vi "inverseKinematicsCode.vi"(8 "Z":dbl, 9 "Y":dbl, 10 "X":dbl) -> (0 "THETA3":dbl, 1 "THETA2":dbl, 2 "THETA1":dbl)   [LabVIEW 2020]
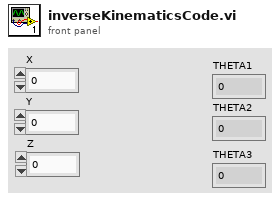
[diagram p1: front panel]
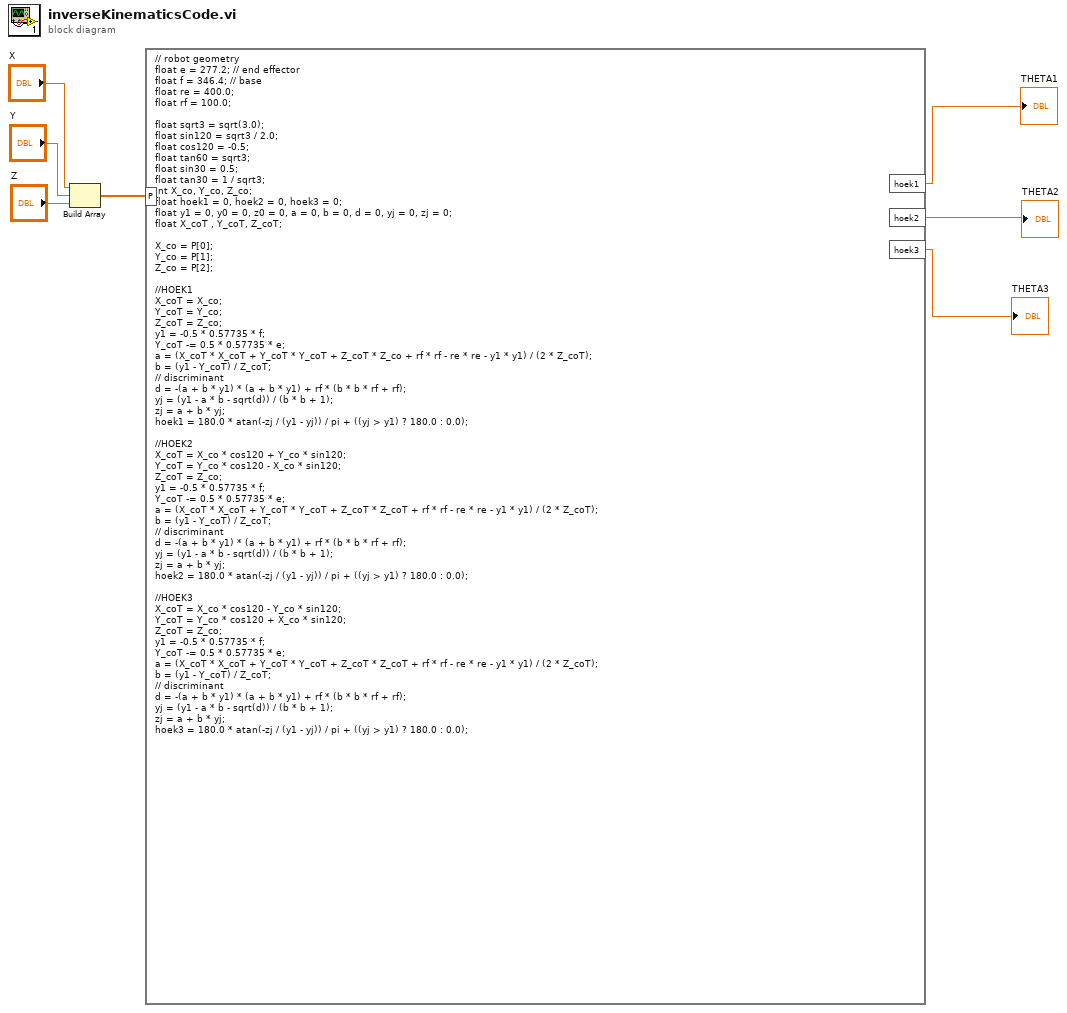
[diagram p0: block diagram]
diagram:
  n1 = Build Array("X", "Y", "Z") -> (w7:dbl[])
  n2 = formula code="// robot geometry\nfloat e = 277.2; // end effector\nfloat f = 346.4; // base\nfloat re = 400.0;\nfloat rf = 100.0;\n\nfloat sqrt3 = sqrt(3.0);\nfloat sin120 = sqrt3 / 2.0;\nfloat cos120 = -0.5;\nfloat tan60 = sqrt3;\nfloat sin30 = 0.5;\nfloat tan30 = 1 / sqrt3;\nint X_co, Y_co, Z_co;\nfloat hoek1 = 0, hoek2 = 0, hoek3 = 0;\nfloat y1 = 0, y0 = 0, z0 = 0, a = 0, b = 0, d = 0, yj = 0, zj = 0;\nfloat X_coT , Y_coT, Z_coT;\n\nX_co = P[0];\nY_co = P[1];\nZ_co = P[2];\n\n//HOEK1\nX_coT = X_co;\nY_coT = Y_co; \nZ_coT = Z_co;\ny1 = -0.5 * 0.57735 * f;\nY_coT -= 0.5 * 0.57735 * e;\na = (X_coT * X_coT + Y_coT * Y_coT + Z_coT * Z_co + rf * rf - re * re - y1 * y1) / (2 * Z_coT);\nb = (y1 - Y_coT) / Z_coT;\n// discriminant\nd = -(a + b * y1) * (a + b * y1) + rf * (b * b * rf + rf);\nyj = (y1 - a * b - sqrt(d)) / (b * b + 1);\nzj = a + b * yj;\nhoek1 = 180.0 * atan(-zj / (y1 - yj)) / pi + ((yj > y1) ? 180.0 : 0.0);\n\n//HOEK2\nX_coT = X_co * cos120 + Y_co * sin120;\nY_coT = Y_co * cos120 - X_co * sin120;\nZ_coT = Z_co;\ny1 = -0.5 * 0.57735 * f;\nY_coT -= 0.5 * 0.57735 * e;\na = (X_coT * X_coT + Y_coT * Y_coT + Z_coT * Z_coT + rf * rf - re * re - y1 * y1) / (2 * Z_coT);\nb = (y1 - Y_coT) / Z_coT;\n// discriminant\nd = -(a + b * y1) * (a + b * y1) + rf * (b * b * rf + rf);\nyj = (y1 - a * b - sqrt(d)) / (b * b + 1);\nzj = a + b * yj;\nhoek2 = 180.0 * atan(-zj / (y1 - yj)) / pi + ((yj > y1) ? 180.0 : 0.0);\n\n//HOEK3\nX_coT = X_co * cos120 - Y_co * sin120;\nY_coT = Y_co * cos120 + X_co * sin120;\nZ_coT = Z_co;\ny1 = -0.5 * 0.57735 * f;\nY_coT -= 0.5 * 0.57735 * e;\na = (X_coT * X_coT + Y_coT * Y_coT + Z_coT * Z_coT + rf * rf - re * re - y1 * y1) / (2 * Z_coT);\nb = (y1 - Y_coT) / Z_coT;\n// discriminant\nd = -(a + b * y1) * (a + b * y1) + rf * (b * b * rf + rf);\nyj = (y1 - a * b - sqrt(d)) / (b * b + 1);\nzj = a + b * yj;\nhoek3 = 180.0 * atan(-zj / (y1 - yj)) / pi + ((yj > y1) ? 180.0 : 0.0);"("P"=w7) -> ("hoek1"=→"THETA1":dbl, "hoek3"=→"THETA3":dbl, "hoek2"=→"THETA2":dbl)
